vi "BRig_Host_v0,54.vi"() -> ()   [LabVIEW 2014]
uses:
  <vilib>/WebDAVClient/Advanced/SessionHandle.ctl
  BRig_Host__global__stopHost.vi
  <vilib>/Utility/file.llb/Write To Spreadsheet File (DBL).vi
  <vilib>/WebDAVClient/NI_WebDAV.lvlib
panel:
  out "output_dataTS":u16[][](array[numeric])
  out "output_dataPlot":u16[][](array[numeric])
  out "DAB_nTimeout":u16 caption="# Rewards in Current Block"
  out "FreeReward_c_R":u16
  out "FreeReward_c_L":u16
  out "BTPR_avg_R":dbl
  out "T2R_avg_R":dbl
  out "BTPR_avg_L":dbl
  out "T2R_avg_L":dbl
  out "BTPR_cur":u16
  out "T2R_cur":u16
  out "nReward":u16 caption="# Rewards in Current Block"
  out "BUR_target":u16 caption="Target Trials Per Block"
  out "nTrial":u16
  out "nReward_Right":u16 caption="# Rewards Total (Right)"
  out "nReward_Left":u16 caption="# Rewards Total (Left)"
  out "nReward_cur":u16 caption="# Rewards in Current Block"
  out "TpB_target":u16 caption="Target Trials Per Block"
  out "iBlock":u16 caption="Current Block"
  out "iTrial":u16 caption="Current Trial"
  out "DAB_nRewards_ProbLow_percent":u16 caption="# Rewards Total (Right)"
  out "DAB_nRewards_ProbHigh_percent":u16 caption="# Rewards Total (Left)"
  out "DAB_nRewards_ProbLow":u16 caption="# Rewards Total (Right)"
  out "DAB_nRewards_ProbHigh":u16 caption="# Rewards Total (Left)"
  out "DAB_nRewards_total":u16 caption="# Rewards in Current Block"
  out "DAB_nTrial":u16
  out "DAB_nRewards_Right":u16 caption="# Rewards Total (Right)"
  out "DAB_nRewards_Left":u16 caption="# Rewards Total (Left)"
  out "writeError":bool
  out "error IO":errorcluster
  out "error_loopP_loadSettings":errorcluster caption="error out"
  out "testCmdList":u16[][](array[numeric])
  in  "ClosedLoop":bool
  in  "module":string=" module1 "
  in  "input_updateTrial_subsequent":u16
  in  "input_updateTrial_first":u16
  in  "input_forceUpdate":bool
  in  "ClosedLoop":u16[](array[numeric])
  in  "testNewLaserSettings":bool
  in  "LoadSettings":bool
  in  "DisplayNumber":u16
  out "XY Graph":cluster{u16[], u16[]}[](graph)
  in  "threshold_2":u16=600
  in  "threshold_1":u16=300
  in  "Port (F=A/B, T=C)":bool
  out "I_ExpRun":bool
  out "TCP_connection":bool
  in  "stopHost":bool
  # "# Trials Displayed\n( 0 = all )"
  # "Selection\nTime Thresholds"
  # "Dual Armed Bandit"
  # "Standard or 2 Cues"
  # "Total"
  # "# Trials"
  # "# Rewards"
  # "Block Target"
  # "# Blocks"
  # "# Trials"
  # "# Rewards"
  # "Left           Right"
  # "Bad Trials\nPost Reward"
  # "Trials 2 Reward"
  # "# Timeouts"
  # "Block"
  # "# Trials"
  # "# Rewards"
  # "Current\nBlock"
  # "# Selections"
  # "High Prob    Low Prob"
  # "avg L"
  # "Total"
  # "# Rewards"
  # "# Trials"
  # "avg R"
  # "% Selections"
  # "High Prob    Low Prob"
  # "FreeRewards"
  # "Left           Right"
  # "Unknown"
  # "reward1"
  # "reward2"
  # "reward3"
  # "wrong1"
  # "wrong2"
  # "wrong3"
  # "timeout"
  # "trig1"
  # "trig2"
  # "Port Switch\nToggle TRUE if debugging"
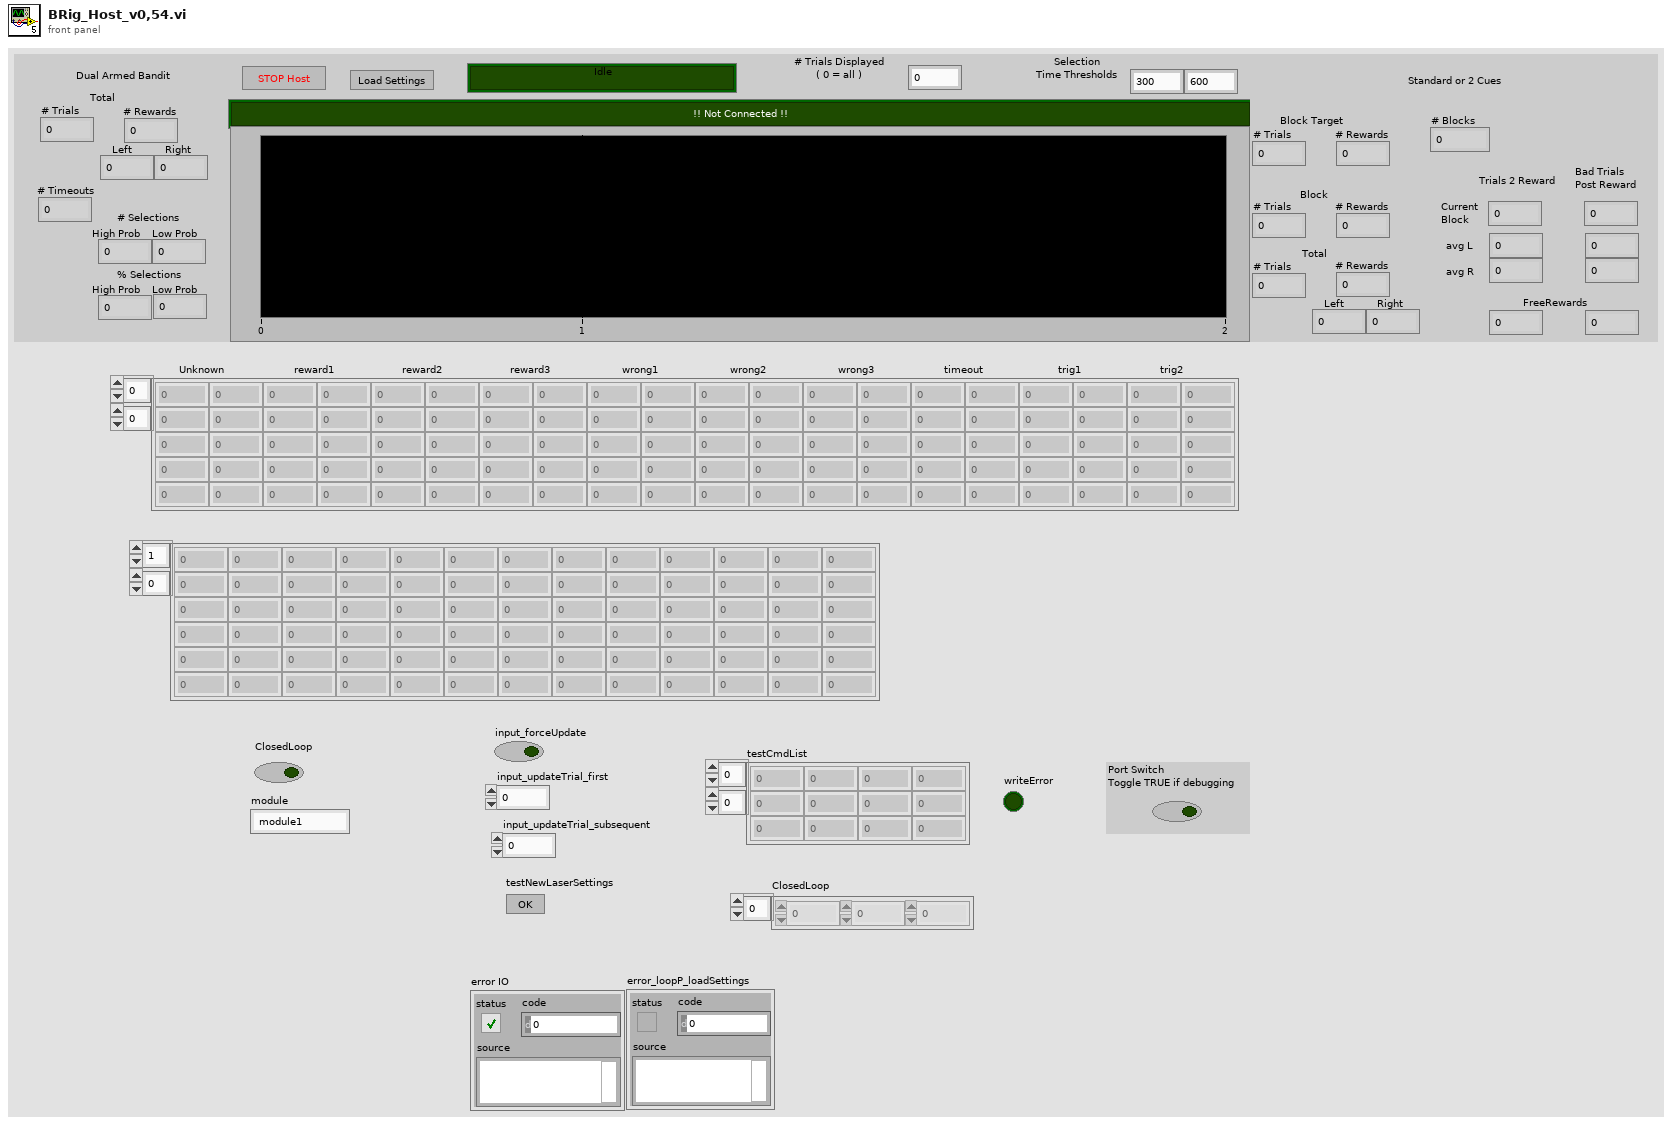
[diagram p1: front panel]
types:
  T1 = typedef "NI_WebDAV.lvlib/SessionHandle.ctl" = refnum<k1>
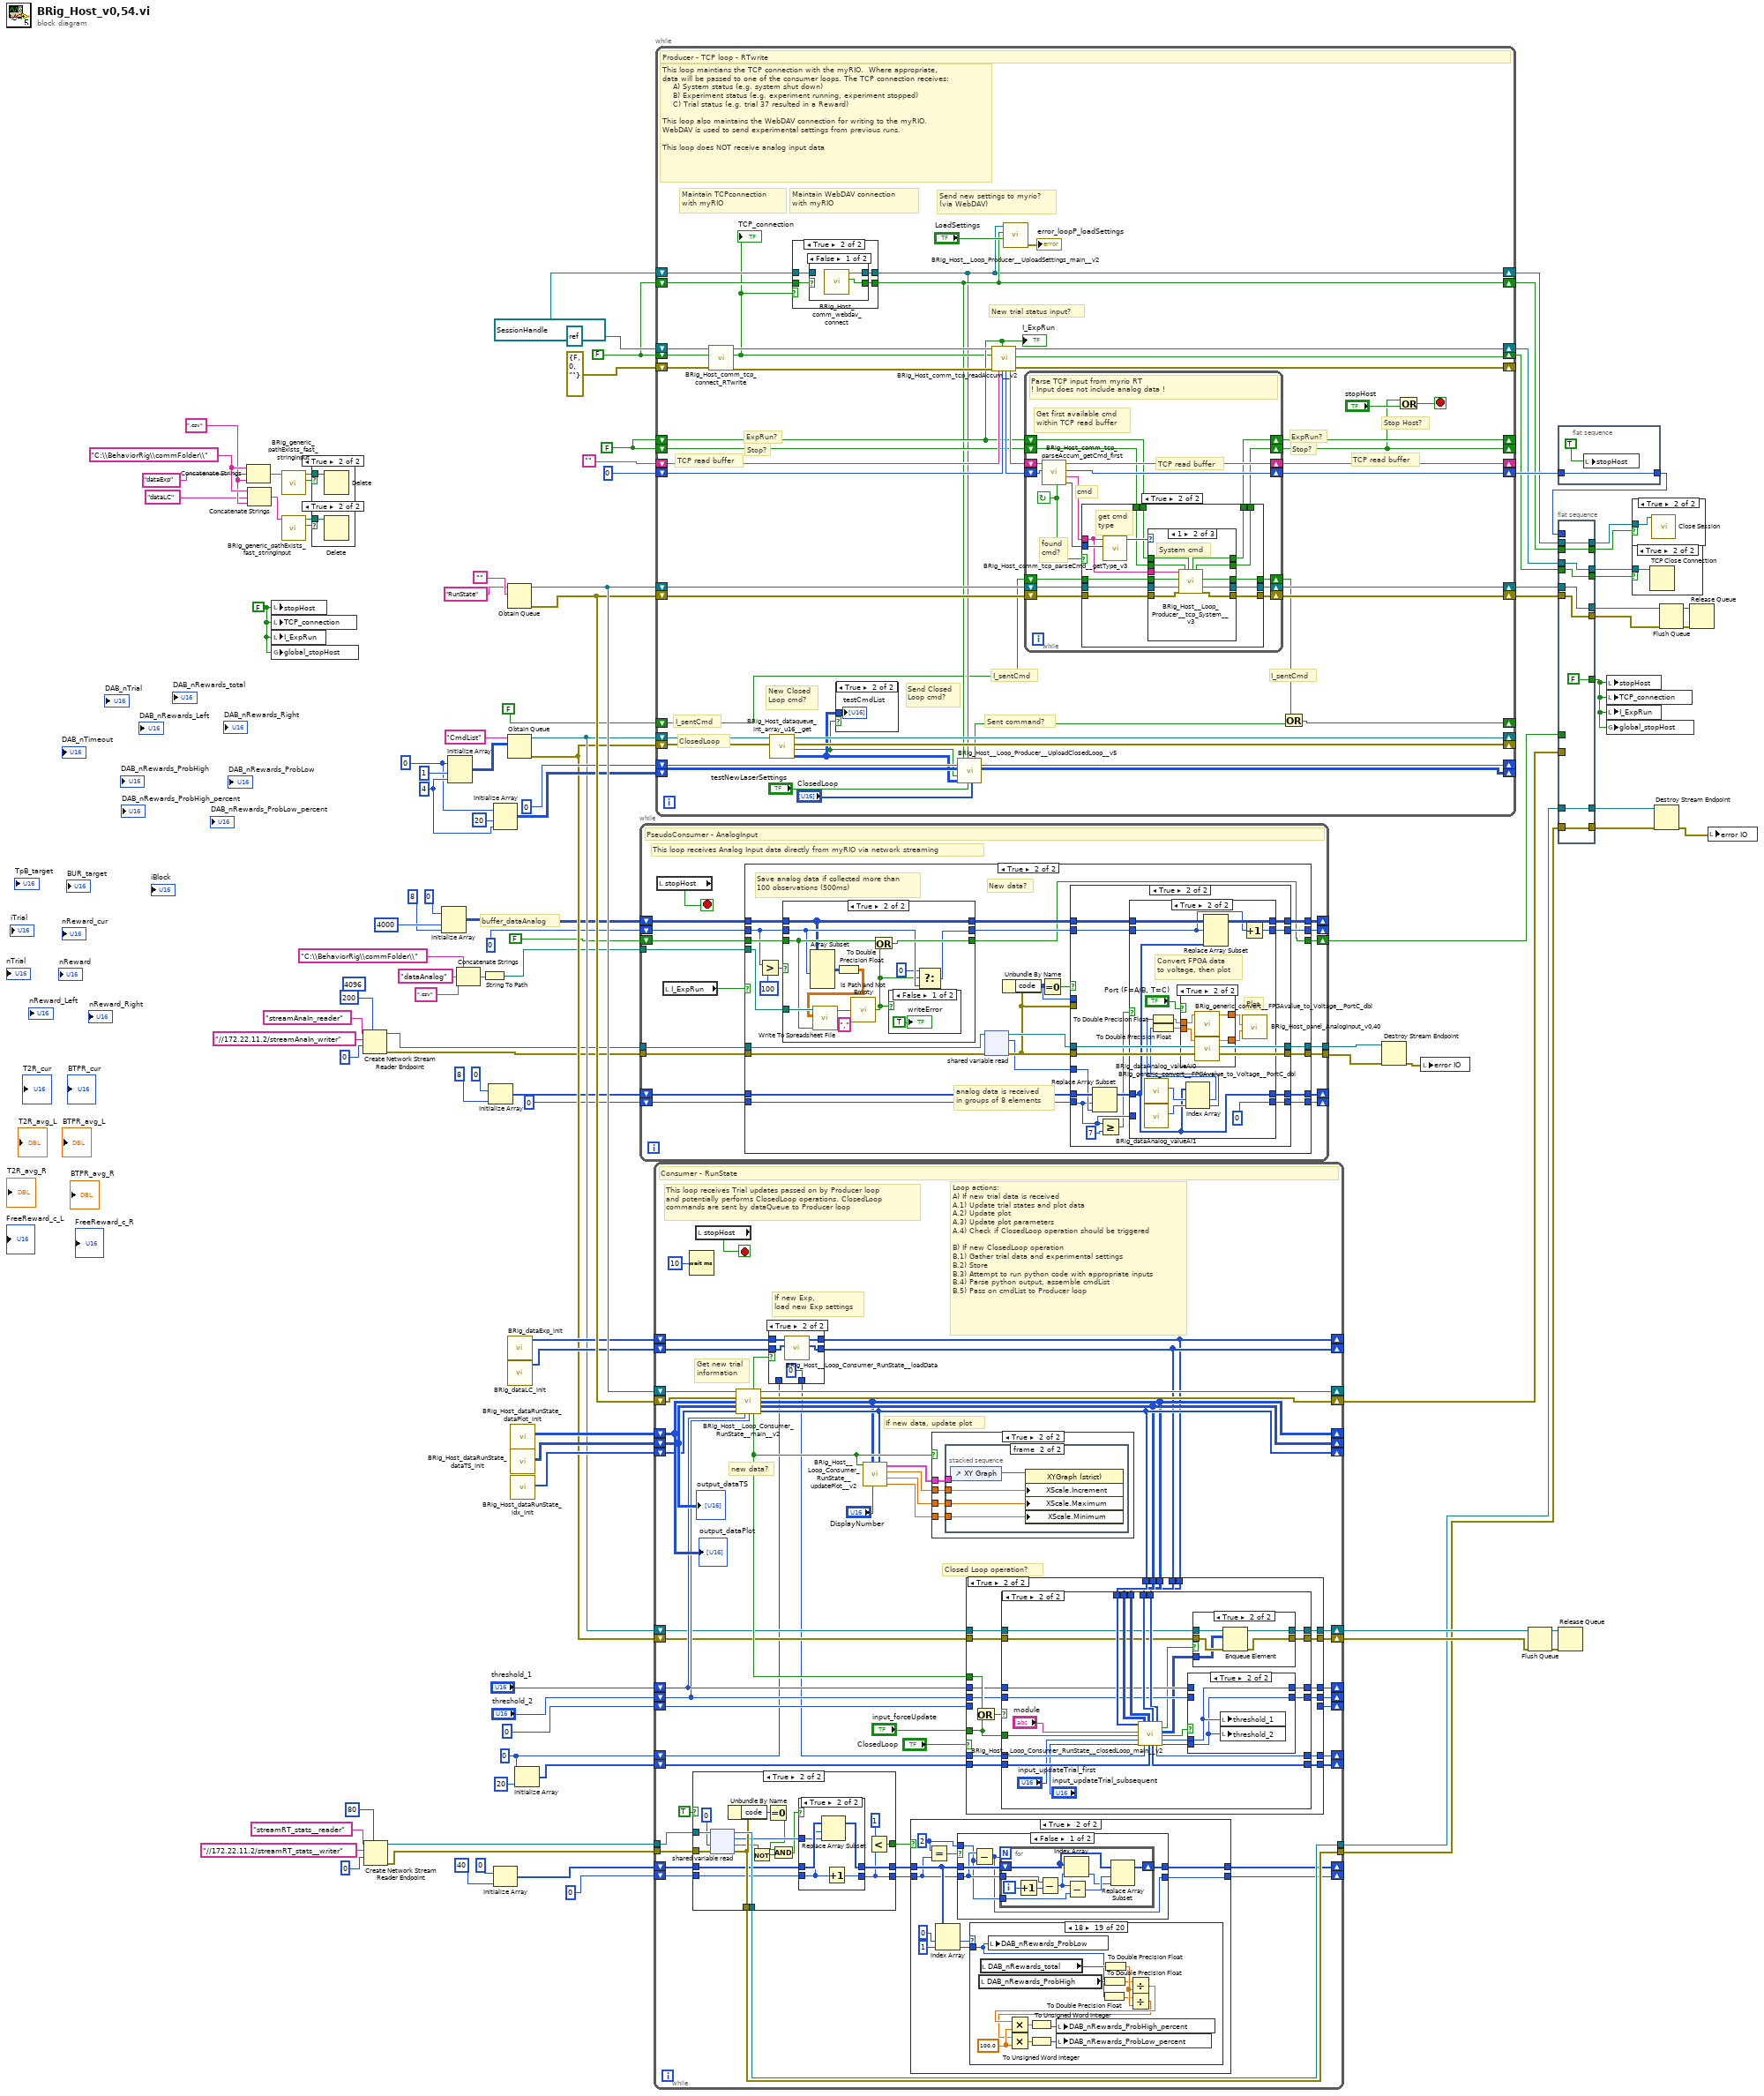
[diagram p0: block diagram]
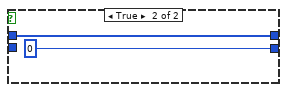
[diagram p9: hidden frame]
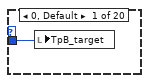
[diagram p10: hidden frame]
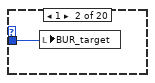
[diagram p11: hidden frame]
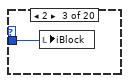
[diagram p12: hidden frame]
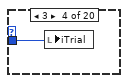
[diagram p13: hidden frame]
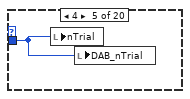
[diagram p14: hidden frame]
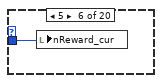
[diagram p15: hidden frame]
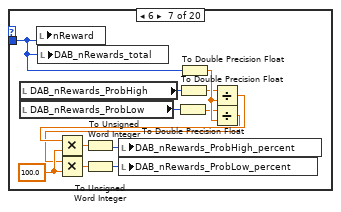
[diagram p16: hidden frame]
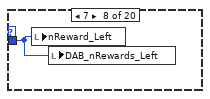
[diagram p17: hidden frame]
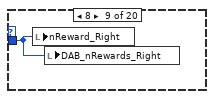
[diagram p18: hidden frame]
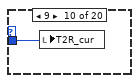
[diagram p19: hidden frame]
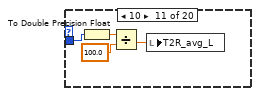
[diagram p20: hidden frame]
diagram:
  (unwired) 4096 ("reader buffer size")
  w41 = u16 0 ("element")
  w42 = 4 ("dimension size")
  w58 = u16 0
  w70 = ".csv" ("string")
  w71 = "C:\\BehaviorRig\\commFolder\\"
  w83 = T1 refnum items=["Session NI_WebDAV"] ("session handle")
  w101 = FALSE ("stopHost")
  w102 = FALSE
  w84 = FALSE
  # "buffer_dataAnalog"
  n1 = Concatenate Strings(w71, "dataExp" ("string"), w70) -> (w65:string)
  n2 = Concatenate Strings(w71, "dataLC" ("string"), w70) -> (w62:string)
  n3 = local write "stopHost"(w101) -> ()
  n4 = local write "TCP_connection"(w101) -> ()
  n5 = local write "I_ExpRun"(w101) -> ()
  n6 = global write "BRig_Host__global__stopHost.vi" "global_stopHost"(w101) -> ()
  n7 = call "BRig_generic_pathExists_fast_stringInput.vi"("input_filePath"=w65) -> ("output_Iexist"=w67:bool, "output_filePath"=w66:path)  [unwired: 8 in, 1 out]
  n8 = call "BRig_generic_pathExists_fast_stringInput.vi"("input_filePath"=w62) -> ("output_Iexist"=w63:bool, "output_filePath"=w64:path)  [unwired: 8 in, 1 out]
  n9 = case shown="True" w67 {
    tunnel: w66 -> [_ w107]
    frame False {
    }
    frame True {
      n10 = Delete(path (use dialog)=w107) -> ()  [unwired: 4 in, 3 out]
    }
  }
  n11 = case shown="True" w63 {
    tunnel: w64 -> [_ w108]
    frame False {
    }
    frame True {
      n12 = Delete(path (use dialog)=w108) -> ()  [unwired: 4 in, 3 out]
    }
  }
  n13 = Create Network Stream Reader Endpoint(7:200 ("reader buffer size"), 9:u16 0 ("element"), 10:"//172.22.11.2/streamAnaIn_writer" ("writer url"), 11:"streamAnaIn_reader" ("reader name")) -> (0:w25:errorcluster, 3:w26:refnum<k21>)  [unwired: 3 in]
  n14 = Create Network Stream Reader Endpoint(7:80 ("reader buffer size"), 9:u16 0 ("element"), 10:"//172.22.11.2/streamRT_stats__writer" ("writer url"), 11:"streamRT_stats__reader" ("reader name")) -> (0:w11:errorcluster, 3:w12:refnum<k21>)  [unwired: 3 in]
  n15 = Initialize Array(u16 0 ("element"), 4000 ("dimension size"), 8 ("dimension size")) -> (w37:u16[][])
  n16 = Initialize Array(w41, 1 ("dimension size"), w42) -> (w53:u16[][])
  n17 = Concatenate Strings("C:\\BehaviorRig\\commFolder\\" ("string"), "dataAnalog" ("input_filename"), ".csv" ("string")) -> (w34:string)
  n18 = String To Path(string=w34) -> (path=w31:path)
  n19 = Initialize Array(u16 0 ("element"), 8 ("dimension size")) -> (w18:u16[])
  n20 = Initialize Array(w41, 20 ("dimension size"), w42) -> (w72:u16[][])
  n21 = Initialize Array(u16 0 ("element"), 40 ("dimension size")) -> (w8:u16[])
  n22 = Obtain Queue(name (unnamed)="RunState", element data type="") -> (queue out=w93:refnum<queue>, error out=w92:errorcluster)  [unwired: 3 in, 1 out]
  n23 = Obtain Queue(name (unnamed)="CmdList", element data type=w53) -> (queue out=w52:refnum<queue>, error out=w51:errorcluster)  [unwired: 3 in, 1 out]
  n24 = call "BRig_dataExp_init.vi"() -> ("output_dataExp"=w61:u16[])  [unwired: 11 in]
  n25 = call "BRig_dataLC_init.vi"() -> ("output_dataLC"=w60:u16[])  [unwired: 11 in]
  n26 = call "BRig_Host_dataRunState_dataPlot_init.vi"() -> ("output_dataPlot"=w89:u16[][])  [unwired: 11 in]
  n27 = call "BRig_Host_dataRunState_dataTS_init.vi"() -> ("output_dataTS"=w88:u16[][])  [unwired: 11 in]
  n28 = call "BRig_Host_dataRunState_idx_init.vi"() -> ("output_idx"=w87:i32[])  [unwired: 11 in]
  n29 = Initialize Array(w58, 20 ("dimension size")) -> (w56:u16[])
  n30 = while {
    shift-right: [w123] -> _
    shift-left: w37 -> [w125]
    shift-right: [w122] -> _
    shift-left: 0 -> [w124]
    tunnel: w31 -> [w121]
    shift-right: [w119] -> w29
    shift-left: FALSE -> [w120]
    tunnel: w26 -> [w117]
    tunnel: w25 -> [w116]
    tunnel: [w115] -> w23
    tunnel: [w114] -> w22
    shift-right: [w111] -> _
    shift-left: w18 -> [w113]
    shift-right: [w110] -> _
    shift-left: 0 ("element") -> [w112]
    stop <- w109 stop-if-true
    # "This loop receives Analog Input data directly from myRIO via network streaming"
    # "PseudoConsumer - AnalogInput"
    n31 = local read "stopHost"() -> (w109:bool)
    n32 = local read "I_ExpRun"() -> (w118:bool)
    n33 = case shown="True" w118 {
      tunnel: w125 -> [w132 w156]
      tunnel: w124 -> [_ w142]
      tunnel: [w132 w151] -> w123
      tunnel: [0 w149] -> w122
      tunnel: w121 -> [_ w154]
      tunnel: w120 -> [_ w155]
      tunnel: [FALSE w139] -> w119
      tunnel: w117 -> [w129 w148]
      tunnel: w116 -> [w128 w147]
      tunnel: [w129 w145] -> w115
      tunnel: [w128 w143] -> w114
      tunnel: w113 -> [w127 w137]
      tunnel: w112 -> [_ w136]
      tunnel: [w127 w135] -> w111
      tunnel: [0 ("element") w134] -> w110
      frame False {
        n34 = Wait (ms)(milliseconds to wait=u32 20) -> ()  [unwired: 1 out]
      }
      frame True {
        # "analog data is received\nin groups of 8 elements"
        # "New data?"
        # "Save analog data if collected more than\n100 observations (500ms)"
        n35 = Greater?(x=w142, y=100) -> (0:w157:bool)
        n36 = case shown="True" w157 {
          tunnel: w156 -> [w216 w219]
          tunnel: [w216 w219] -> w152
          tunnel: w142 -> [w215 w221]
          tunnel: w155 -> [w214 w223]
          tunnel: [w215 w220] -> w150
          tunnel: [w214 w222] -> w139
          tunnel: w154 -> [_ w228]
          frame False {
          }
          frame True {
            n37 = Array Subset(array=w219, length (row)=w221) -> (w227:u16[][])  [unwired: 3 in]
            n38 = To Double Precision Float(number=w227) -> (double precision float=w226:dbl[][])
            n39 = call-poly <vilib>:"Write To Spreadsheet File.vi"("delimiter (\\t)"="," ("delimiter (\\t)"), "append to file? (new file:F)"=w223, "2D data"=w226, "file path (dialog if empty)"=w228) -> ("new file path (Not A Path if cancelled)"=w224:path)  [unwired: 4 in]
            n40 = call <vilib>:"Is Path and Not Empty.vi"("path"=w224) -> ("Is Path and Not Empty?"=w217:bool)  [unwired: 4 in]
            n41 = Or(x=w223, y=w217) -> (x .or. y?=w222:bool)
            n42 = case shown="False" w217 {
              frame False {
                "writeError" <- TRUE ("writeError")
              }
              frame True {
              }
            }
            n43 = Select(t=0, s=w217, f=w221) -> (s? t:f=w220:i32)
          }
        }
        n44 = shared-variable-read(w148, w147) -> (w146:refnum<k21>, w144:errorcluster, w138:u16)  [unwired: 1 in, 1 out]
        n45 = Unbundle By Name(w144) -> ("code"=w140:i32)
        n46 = Equal To 0?(x=w140) -> (x = 0?=w153:bool)
        n47 = case shown="True" w153 {
          tunnel: w152 -> [w170 w185]
          tunnel: [w170 w184] -> w151
          tunnel: w150 -> [w169 w183]
          tunnel: [w169 w182] -> w149
          tunnel: w144 -> [w167 _]
          tunnel: w146 -> [w166 w181]
          tunnel: [w166 w181] -> w145
          tunnel: w144 -> [w165 w180]
          tunnel: [w165 w180] -> w143
          tunnel: w140 -> [w164 _]
          tunnel: w138 -> [_ w178]
          tunnel: w137 -> [w159 w179]
          tunnel: w136 -> [w158 w176]
          tunnel: [w159 w173] -> w135
          tunnel: [w158 w175] -> w134
          frame False {
            n48 = Equal?(x=-314100, y=w164) -> (x = y?=w162:bool)
            n49 = Equal?(x=-314220, y=w164) -> (x = y?=w161:bool)
            n50 = Or(x=w162, y=w161) -> (x .or. y?=w160:bool)
            n51 = case shown="False" w160 {
              tunnel: w167 -> [w171 _]
              frame False {
                "error IO" <- w171
              }
              frame True {
              }
            }
          }
          frame True {
            n52 = Replace Array Subset(array=w179, new element=w178, index=w176) -> (w174:u16[])
            n53 = Greater Or Equal?(x=w176, y=7) -> (x >= y?=w172:bool)
            n54 = case shown="True" w172 {
              tunnel: w185 -> [w190 w205]
              tunnel: [w190 w204] -> w184
              tunnel: w183 -> [w189 w203]
              tunnel: [w189 w202] -> w182
              tunnel: w176 -> [w188 _]
              tunnel: [w187 0 ("y")] -> w175
              tunnel: w174 -> [w186 w193]
              tunnel: [w186 w193] -> w173
              frame False {
                n55 = Increment(x=w188) -> (x+1=w187:i32)
              }
              frame True {
                # "Convert FPGA data\nto voltage, then plot"
                # "Plot"
                n56 = call "BRig_dataAnalog_valueAI0.vi"() -> ("output_valueAI0"=w195:i32)  [unwired: 11 in]
                n57 = call "BRig_dataAnalog_valueAI1.vi"() -> ("output_valueAI1"=w196:i32)  [unwired: 11 in]
                n58 = Index Array(array=w193, index #1=w195, index #2=w196) -> (element #1=w192:u16, element #2=w191:u16)
                n59 = To Double Precision Float(number=w192) -> (double precision float=w197:dbl)
                n60 = To Double Precision Float(number=w191) -> (double precision float=w198:dbl)
                n61 = case shown="True" "Port (F=A/B, T=C)" {
                  tunnel: w197 -> [w207 w213]
                  tunnel: w198 -> [w206 w212]
                  tunnel: [w209 w211] -> w200
                  tunnel: [w208 w210] -> w199
                  frame False {
                    n62 = call "BRig_generic_convert__FPGAvalue_to_Voltage__PortAorB_dbl.vi"("input_FPGAvalue_PortAorB"=w207) -> ("output_voltage"=w209:dbl)  [unwired: 10 in]
                    n63 = call "BRig_generic_convert__FPGAvalue_to_Voltage__PortAorB_dbl.vi"("input_FPGAvalue_PortAorB"=w206) -> ("output_voltage"=w208:dbl)  [unwired: 10 in]
                  }
                  frame True {
                    n64 = call "BRig_generic_convert__FPGAvalue_to_Voltage__PortC_dbl.vi"("input_FPGAvalue_PortC"=w213) -> ("output_voltage"=w211:dbl)  [unwired: 10 in]
                    n65 = call "BRig_generic_convert__FPGAvalue_to_Voltage__PortC_dbl.vi"("input_FPGAvalue_PortC"=w212) -> ("output_voltage"=w210:dbl)  [unwired: 10 in]
                  }
                }
                n66 = Replace Array Subset(array=w205, new element=w193, index (row)=w203) -> (w204:u16[][])  [unwired: 1 in]
                n67 = Increment(x=w203) -> (x+1=w202:i32)
                n68 = call "BRig_Host_panel_AnalogInput_v0,40.vi"("graph_ai1"=w199, "graph_ai0"=w200) -> ()  [unwired: 10 in]
              }
            }
          }
        }
      }
    }
  }
  n69 = while {
    shift-right: [w274] -> _
    shift-left: w93 -> [w275]
    shift-right: [w272] -> w46
    shift-left: w92 -> [w273]
    shift-right: [w255] -> _
    shift-left: w89 -> [w271]
    shift-right: [w256] -> _
    shift-left: w88 -> [w270]
    shift-right: [w257] -> _
    shift-left: w87 -> [w269]
    shift-right: [w265] -> _
    shift-left: "threshold_1" -> [w264]
    shift-right: [w263] -> _
    shift-left: "threshold_2" -> [w262]
    shift-right: [w253] -> _
    shift-left: w61 -> [w267]
    shift-right: [w254] -> _
    shift-left: w60 -> [w266]
    shift-right: [w247] -> _
    shift-left: w58 -> [w245]
    shift-right: [w259] -> _
    shift-left: u8 0 -> [w260]
    shift-right: [w246] -> _
    shift-left: w56 -> [w243]
    shift-right: [w250] -> w48
    shift-left: w52 -> [w252]
    shift-right: [w249] -> w47
    shift-left: w51 -> [w251]
    tunnel: w12 -> [w241]
    tunnel: w11 -> [w240]
    shift-right: [w232] -> _
    shift-left: w8 -> [w237]
    shift-right: [w231] -> _
    shift-left: 0 ("element") -> [w236]
    tunnel: [w239] -> w4
    tunnel: [w238] -> w3
    stop <- w242 stop-if-true
    # "Closed Loop operation?"
    # "Loop actions:\nA) If new trial data is received\nA.1) Update trial states and plot data\nA.2) Update plot\nA.3) Update plot parameters\nA.4) Check if ClosedLoop operation should be triggered\n\nB) If new ClosedLoop operation\nB.1) Gather trial data and experimental settings\nB.2) Store\nB.3) Attempt to run python code with appropriate inputs\nB.4) Parse python output, assemble cmdList\nB.5) Pass on cmdList to Producer loop"
    # "This loop receives Trial updates passed on by Producer loop\nand potentially performs ClosedLoop operations. ClosedLoop\ncommands are sent by dataQueue to Producer loop"
    # "If new data, update plot"
    # "If new Exp,\nload new Exp settings"
    # "new data?"
    # "Get new trial\ninformation"
    # "Consumer - RunState"
    n70 = Wait (ms)(milliseconds to wait=u32 10) -> ()  [unwired: 1 out]
    n71 = case shown="True" TRUE {
      selector: TRUE -> [w282 _]
      tunnel: w241 -> [w286 w302]
      tunnel: w240 -> [w285 w301]
      tunnel: [w286 w300] -> w239
      tunnel: [w285 w299] -> w238
      tunnel: w237 -> [w284 w297]
      tunnel: w236 -> [w283 w296]
      tunnel: [w282 w294] -> w235
      tunnel: [w284 w293] -> w234
      tunnel: [w283 w292] -> w233
      frame False {
      }
      frame True {
        n72 = shared-variable-read(w302, w301, 0 ("timeout ms (-1)")) -> (w300:refnum<k21>, w299:errorcluster, w290:bool, w298:u16)
        n73 = Unbundle By Name(w299) -> ("code"=w303:i32)
        n74 = Not(x=w290) -> (.not. x?=w289:bool)
        n75 = Equal To 0?(x=w303) -> (x = 0?=w288:bool)
        n76 = And(x=w288, y=w289) -> (x .and. y?=w287:bool)
        n77 = case shown="True" w287 {
          tunnel: w298 -> [_ w309]
          tunnel: w297 -> [w305 w310]
          tunnel: w296 -> [w304 w308]
          tunnel: [w305 w306] -> w293
          tunnel: [w304 w307] -> w292
          frame False {
          }
          frame True {
            n78 = Replace Array Subset(array=w310, new element=w309, index=w308) -> (w306:u16[])
            n79 = Increment(x=w308) -> (x+1=w307:i32)
          }
        }
        n80 = Less?(x=1, y=w292) -> (x < y?=w294:bool)
      }
    }
    n81 = local read "stopHost"() -> (w242:bool)
    n82 = call "BRig_Host__Loop_Consumer_RunState__main__v2.vi"("input_hDataQueue"=w275, "input_errorDataQueue"=w273, "input_dataPlot"=w271, "input_dataTS"=w270, "input_idx"=w269, "threshold_1"=w264, "threshold_2"=w262) -> ("output_ExpStart"=w268:bool, "output_hDataQueue"=w274:refnum<queue>, "output_errorDataQueue"=w272:errorcluster, "output_dataPlot"=w255:u16[][], "output_dataTS"=w256:u16[][], "output_updatePlot"=w258:bool, "output_idx"=w257:i32[])  [unwired: 2 in]
    n83 = case shown="True" w268 {
      tunnel: w267 -> [w490 w492]
      tunnel: [w490 w495] -> w253
      tunnel: w266 -> [w489 w493]
      tunnel: [w489 w494] -> w254
      tunnel: w245 -> [w488 _]
      tunnel: [w488 u16 0] -> w244
      frame False {
      }
      frame True {
        n84 = call "BRig_Host__Loop_Consumer_RunState__loadData.vi"("input_dataLC"=w493, "input_dataExp"=w492) -> ("output_dataLC"=w494:u16[], "output_dataExp"=w495:u16[])  [unwired: 8 in]
      }
    }
    n85 = call "BRig_Host__Loop_Consumer_RunState__updatePlot__v2.vi"("input_idx"=w257, "input_DisplayNumber"="DisplayNumber", "input_dataPlot"=w255, "input_updatePlot"=w258) -> ("output_X_min"=w278:dbl, "output_X_max"=w277:dbl, "output_X_inc"=w276:dbl, "XY Graph"=w279:cluster{u16[], u16[]}[])  [unwired: 4 in]
    n86 = case shown="True" w235 {
      tunnel: w234 -> [w312 w317]
      tunnel: w233 -> [w311 w315]
      tunnel: [w312 w316] -> w232
      tunnel: [w311 w314] -> w231
      frame False {
      }
      frame True {
        w313 = 2 ("x")
        n87 = Equal?(x=w313, y=w315) -> (x = y?=w318:bool)
        n88 = Index Array(array=w317, index #1=0 ("index"), index #2=1 ("index")) -> (element #1=w320:u16, element #2=w319:u16)
        n89 = case shown="False" w318 {
          tunnel: w317 -> [w327 w338]
          tunnel: [w323 w338] -> w316
          tunnel: w315 -> [w326 _]
          tunnel: [w324 0 ("index")] -> w314
          tunnel: w313 -> [w325 _]
          frame False {
            n90 = Subtract(x=w326, y=w325) -> (x-y=w324:i32)
            n91 = for {
              N: w324 -> [_]
              shift-right: [w328] -> w323
              shift-left: w327 -> [w331]
              tunnel: w326 -> [w334]
              tunnel: w325 -> [w333]
              i -> [w336]
              n92 = Increment(x=w336) -> (x+1=w335:i32)
              n93 = Subtract(x=w334, y=w335) -> (x-y=w332:i32)
              n94 = Index Array(array=w331, index=w332) -> (element=w329:u16)
              n95 = Subtract(x=w332, y=w333) -> (x-y=w330:i32)
              n96 = Replace Array Subset(array=w331, new element=w329, index=w330) -> (w328:u16[])
            }
          }
          frame True {
          }
        }
        n97 = case shown="18" w320 {
          tunnel: w319 -> [w339 w340 w341 w342 w343 w344 w352 w358 w359 w360 w364 w368 w369 w371 w375 w378 w379 w380 w393 w406]
          frame 0, Default {
            n98 = local write "TpB_target"(w339) -> ()
          }
          frame 1 {
            n99 = local write "BUR_target"(w340) -> ()
          }
          frame 2 {
            n100 = local write "iBlock"(w341) -> ()
          }
          frame 3 {
            n101 = local write "iTrial"(w342) -> ()
          }
          frame 4 {
            n102 = local write "nTrial"(w343) -> ()
            n103 = local write "DAB_nTrial"(w343) -> ()
          }
          frame 5 {
            n104 = local write "nReward_cur"(w344) -> ()
          }
          frame 6 {
            w351 = 100.0 ("y")
            n105 = local read "DAB_nRewards_ProbHigh"() -> (w353:u16)
            n106 = local read "DAB_nRewards_ProbLow"() -> (w354:u16)
            n107 = local write "nReward"(w352) -> ()
            n108 = local write "DAB_nRewards_total"(w352) -> ()
            n109 = To Double Precision Float(number=w354) -> (double precision float=w356:dbl)
            n110 = To Double Precision Float(number=w353) -> (double precision float=w355:dbl)
            n111 = To Double Precision Float(number=w352) -> (double precision float=w357:dbl)
            n112 = Divide(x=w355, y=w357) -> (x/y=w350:dbl)
            n113 = Multiply(x=w350, y=w351) -> (x*y=w348:dbl)
            n114 = To Unsigned Word Integer(number=w348) -> (unsigned 16bit integer=w346:u16)
            n115 = local write "DAB_nRewards_ProbHigh_percent"(w346) -> ()
            n116 = Divide(x=w356, y=w357) -> (x/y=w349:dbl)
            n117 = Multiply(x=w349, y=w351) -> (x*y=w347:dbl)
            n118 = To Unsigned Word Integer(number=w347) -> (unsigned 16bit integer=w345:u16)
            n119 = local write "DAB_nRewards_ProbLow_percent"(w345) -> ()
          }
          frame 7 {
            n120 = local write "nReward_Left"(w358) -> ()
            n121 = local write "DAB_nRewards_Left"(w358) -> ()
          }
          frame 8 {
            n122 = local write "nReward_Right"(w359) -> ()
            n123 = local write "DAB_nRewards_Right"(w359) -> ()
          }
          frame 9 {
            n124 = local write "T2R_cur"(w360) -> ()
          }
          frame 10 {
            n125 = To Double Precision Float(number=w364) -> (double precision float=w363:dbl)
            n126 = Divide(x=w363, y=100.0) -> (x/y=w361:dbl)
            n127 = local write "T2R_avg_L"(w361) -> ()
          }
          frame 11 {
            n128 = To Double Precision Float(number=w368) -> (double precision float=w367:dbl)
            n129 = Divide(x=w367, y=100.0) -> (x/y=w365:dbl)
            n130 = local write "T2R_avg_R"(w365) -> ()
          }
          frame 12 {
            n131 = local write "BTPR_cur"(w369) -> ()
          }
          frame 13 {
            n132 = To Double Precision Float(number=w371) -> (double precision float=w373:dbl)
            n133 = Divide(x=w373, y=100.0) -> (x/y=w370:dbl)
            n134 = local write "BTPR_avg_L"(w370) -> ()
          }
          frame 14 {
            n135 = To Double Precision Float(number=w375) -> (double precision float=w376:dbl)
            n136 = Divide(x=w376, y=100.0) -> (x/y=w374:dbl)
            n137 = local write "BTPR_avg_R"(w374) -> ()
          }
          frame 15 {
            n138 = local write "FreeReward_c_L"(w378) -> ()
          }
          frame 16 {
            n139 = local write "FreeReward_c_R"(w379) -> ()
          }
          frame 17 {
            w388 = 100.0 ("y")
            n140 = local read "DAB_nRewards_ProbLow"() -> (w389:u16)
            n141 = local read "DAB_nRewards_total"() -> (w381:u16)
            n142 = local write "DAB_nRewards_ProbHigh"(w380) -> ()
            n143 = To Double Precision Float(number=w389) -> (double precision float=w391:dbl)
            n144 = To Double Precision Float(number=w380) -> (double precision float=w390:dbl)
            n145 = To Double Precision Float(number=w381) -> (double precision float=w392:dbl)
            n146 = Divide(x=w390, y=w392) -> (x/y=w387:dbl)
            n147 = Multiply(x=w387, y=w388) -> (x*y=w385:dbl)
            n148 = To Unsigned Word Integer(number=w385) -> (unsigned 16bit integer=w383:u16)
            n149 = local write "DAB_nRewards_ProbHigh_percent"(w383) -> ()
            n150 = Divide(x=w391, y=w392) -> (x/y=w386:dbl)
            n151 = Multiply(x=w386, y=w388) -> (x*y=w384:dbl)
            n152 = To Unsigned Word Integer(number=w384) -> (unsigned 16bit integer=w382:u16)
            n153 = local write "DAB_nRewards_ProbLow_percent"(w382) -> ()
          }
          frame 18 {
            w401 = 100.0 ("y")
            n154 = local read "DAB_nRewards_ProbHigh"() -> (w402:u16)
            n155 = local read "DAB_nRewards_total"() -> (w394:u16)
            n156 = local write "DAB_nRewards_ProbLow"(w393) -> ()
            n157 = To Double Precision Float(number=w393) -> (double precision float=w404:dbl)
            n158 = To Double Precision Float(number=w402) -> (double precision float=w403:dbl)
            n159 = To Double Precision Float(number=w394) -> (double precision float=w405:dbl)
            n160 = Divide(x=w403, y=w405) -> (x/y=w400:dbl)
            n161 = Multiply(x=w400, y=w401) -> (x*y=w398:dbl)
            n162 = To Unsigned Word Integer(number=w398) -> (unsigned 16bit integer=w396:u16)
            n163 = local write "DAB_nRewards_ProbHigh_percent"(w396) -> ()
            n164 = Divide(x=w404, y=w405) -> (x/y=w399:dbl)
            n165 = Multiply(x=w399, y=w401) -> (x*y=w397:dbl)
            n166 = To Unsigned Word Integer(number=w397) -> (unsigned 16bit integer=w395:u16)
            n167 = local write "DAB_nRewards_ProbLow_percent"(w395) -> ()
          }
          frame 19 {
            n168 = local write "DAB_nTimeout"(w406) -> ()
          }
        }
      }
    }
    n169 = case shown="True" w258 {
      tunnel: w279 -> [_ w499]
      tunnel: w278 -> [_ w498]
      tunnel: w277 -> [_ w497]
      tunnel: w276 -> [_ w496]
      frame False {
      }
      frame True {
        n170 = stacked-sequence {
          tunnel: w499 -> [w500 _]
          tunnel: w498 -> [_ w503]
          tunnel: w497 -> [_ w502]
          tunnel: w496 -> [_ w501]
          frame #0 {
            "XY Graph" <- w500
          }
          frame #1 {
            n171 = control-ref of="XY Graph"() -> (w504:refnum<vi>)
            n172 = property class="XYGraph (strict)"(reference=w504, "XScale.Increment"=w501, "XScale.Maximum"=w502, "XScale.Minimum"=w503) -> ()  [unwired: 1 in, 2 out]
          }
        }
      }
    }
    n173 = case shown="True" "ClosedLoop" {
      tunnel: [w414 w437] -> w265
      tunnel: w264 -> [w415 w438]
      tunnel: [w413 w435] -> w263
      tunnel: w262 -> [w416 w436]
      tunnel: w260 -> [w419 _]
      tunnel: [w412 _] -> w259
      tunnel: w244 -> [w410 w442]
      tunnel: [w410 w440] -> w247
      tunnel: w243 -> [w409 w441]
      tunnel: [w409 w439] -> w246
      tunnel: w258 -> [_ w444]
      tunnel: w257 -> [_ w434]
      tunnel: w256 -> [_ w433]
      tunnel: w255 -> [_ w432]
      tunnel: w254 -> [_ w431]
      tunnel: w253 -> [_ w430]
      tunnel: w252 -> [w408 w429]
      tunnel: w251 -> [w407 w428]
      tunnel: [w408 w427] -> w250
      tunnel: [w407 w426] -> w249
      tunnel: "input_forceUpdate" -> [_ w425]
      frame False {
        n174 = Increment(x=w419) -> (x+1=w411:u8)
        n175 = Less?(x=w411, y=u8 10) -> (x < y?=w417:bool)
        n176 = case shown="False" w417 {
          tunnel: w416 -> [_ w423]
          tunnel: w415 -> [_ w424]
          tunnel: [w421 w424] -> w414
          tunnel: [w420 w423] -> w413
          tunnel: [_ w422] -> w412
          tunnel: w411 -> [_ w422]
          frame False {
            n177 = local read "threshold_1"() -> (w421:u16)
            n178 = local read "threshold_2"() -> (w420:u16)
          }
          frame True {
          }
        }
      }
      frame True {
        n179 = Or(x=w444, y=w425) -> (x .or. y?=w443:bool)
        n180 = case shown="True" w443 {
          tunnel: w425 -> [_ w473]
          tunnel: w442 -> [w450 w476]
          tunnel: w441 -> [w449 w475]
          tunnel: [w450 w469] -> w440
          tunnel: [w449 w470] -> w439
          tunnel: w438 -> [w448 w463]
          tunnel: [w448 w459] -> w437
          tunnel: w436 -> [w447 w462]
          tunnel: [w447 w458] -> w435
          tunnel: w434 -> [_ w468]
          tunnel: w433 -> [_ w467]
          tunnel: w432 -> [_ w466]
          tunnel: w431 -> [_ w465]
          tunnel: w430 -> [_ w464]
          tunnel: w429 -> [w446 w456]
          tunnel: w428 -> [w445 w454]
          tunnel: [w446 w455] -> w427
          tunnel: [w445 w453] -> w426
          frame False {
          }
          frame True {
            n181 = call "BRig_Host__Loop_Consumer_RunState__closedLoop_main__v2.vi"("input_idx"=w468, "input_module"="module", "input_forceUpdate"=w473, "input_updateTrial_first"="input_updateTrial_first", "input_updateTrial_subsequent"="input_updateTrial_subsequent", "input_dataTS"=w467, "input_updateID"=w476, "input_dataPlot"=w466, "input_trialList"=w475, "input_dataLC"=w465, "input_dataExp"=w464) -> ("output_trialList"=w470:u16[], "output_updateID"=w469:u16, 15:"output_cmdList"=w451:bool, 16:"output_cmdList"=w452:u16[][], "output_thres"=w457:bool, "output_thres1"=w461:u16, "output_thres2"=w460:u16)  [unwired: 2 in]
            n182 = case shown="True" w457 {
              tunnel: w463 -> [w485 _]
              tunnel: w462 -> [w484 _]
              tunnel: w461 -> [_ w487]
              tunnel: w460 -> [_ w486]
              tunnel: [w485 w487] -> w459
              tunnel: [w484 w486] -> w458
              frame False {
              }
              frame True {
                n183 = local write "threshold_1"(w487) -> ()
                n184 = local write "threshold_2"(w486) -> ()
              }
            }
            n185 = case shown="True" w451 {
              tunnel: w456 -> [w478 w483]
              tunnel: [w478 w480] -> w455
              tunnel: w454 -> [w477 w482]
              tunnel: [w477 w479] -> w453
              tunnel: w452 -> [_ w481]
              frame False {
              }
              frame True {
                n186 = Enqueue Element(queue=w483, element=w481, error in (no error)=w482) -> (queue out=w480:refnum<queue>, error out=w479:errorcluster)  [unwired: 1 in, 1 out]
              }
            }
          }
        }
      }
    }
    "output_dataPlot" <- w271
    "output_dataTS" <- w270
  }
  n187 = while {
    shift-right: [w531] -> w77
    shift-left: w84 -> [w551]
    shift-right: [w546] -> w78
    shift-left: refnum<k5> refnum ("output_hTCP") -> [w550]
    shift-right: [w545] -> _
    shift-left: errorcluster {"status"=FALSE, "code"=0, "source"=""} ("output_error") -> [w549]
    shift-right: [w540] -> _
    shift-left: "" ("input_strAccum") -> [w544]
    shift-right: [w539] -> w91
    shift-left: 0 ("input_count") -> [w543]
    shift-right: [w538] -> _
    shift-left: w102 -> [w516]
    shift-right: [w514] -> _
    shift-left: w102 -> [w536]
    shift-right: [w533] -> w97
    shift-left: w93 -> [w535]
    shift-right: [w532] -> w96
    shift-left: w92 -> [w534]
    shift-right: [w511] -> w82
    shift-left: w84 -> [w530]
    shift-right: [w510] -> w81
    shift-left: w83 -> [w529]
    shift-right: [w521] -> _
    shift-left: w72 -> [w522]
    shift-right: [w505] -> _
    shift-left: 0 -> [w523]
    shift-right: [w525] -> _
    shift-left: w52 -> [w527]
    shift-right: [w524] -> _
    shift-left: w51 -> [w526]
    shift-right: [w506] -> _
    shift-left: FALSE -> [w509]
    stop <- w513 stop-if-true
    # "ClosedLoop"
    # "TCP read buffer"
    # "TCP read buffer"
    # "I_sentCmd"
    # "Sent command?"
    # "I_sentCmd"
    # "I_sentCmd"
    # "Stop Host?"
    # "Send Closed\nLoop cmd?"
    # "New Closed\nLoop cmd?"
    # "New trial status input?"
    # "ExpRun?"
    # "Stop?"
    # "This loop maintians the TCP connection with the myRIO.  Where appropriate,\ndata will be passed to one of the consumer loops. The TCP connection receives:\n    A) System status (e.g. system shut down)\n    B) Experiment status (e.g. experiment running, experiment stopped)\n    C) Trial status (e.g. trial 37 resulted in a Reward)\n\nThis loop also maintains the WebDAV connection for writing to the myRIO.\nWebDAV is used to send experimental settings from previous runs.\n\nThis loop does NOT receive analog input data"
    # "Send new settings to myrio?\n(via WebDAV)"
    # "ExpRun?"
    # "Stop?"
    # "Maintain TCPconnection\nwith myRIO"
    # "Maintain WebDAV connection\nwith myRIO"
    # "Producer - TCP loop - RTwrite"
    n188 = call "BRig_Host_comm_tcp_connect_RTwrite.vi"("input_error"=w549, "input_connected"=w551, "input_hTCP"=w550) -> ("output_error"=w547:errorcluster, "output_connected"=w515:bool, "output_hTCP"=w548:refnum<k5>)  [unwired: 5 in, 1 out]
    "TCP_connection" <- w515
    n189 = call "BRig_Host_dataqueue_int_array_u16__get.vi"("input_erroDataQueue"=w526, "input_hDataQueue"=w527) -> (0:"output_data"=w518:u16[][], 1:"output_data"=w517:bool, "output_errorDataQueue"=w524:errorcluster, "output_hDataQueue"=w525:refnum<queue>)  [unwired: 6 in]
    n190 = case shown="True" w515 {
      tunnel: w530 -> [w556 w564]
      tunnel: [w555 w563] -> w511
      tunnel: w529 -> [w554 w562]
      tunnel: [w553 w561] -> w510
      frame False {
        n191 = case shown="True" w556 {
          selector: w556 -> [w558 _]
          tunnel: [w558 FALSE] -> w555
          tunnel: w554 -> [w557 w559]
          tunnel: [w557 _] -> w553
          frame False {
          }
          frame True {
            n192 = call <vilib>:"Close Session.vi"("session handle"=w559) -> ()  [unwired: 14 in, 1 out]
          }
        }
      }
      frame True {
        n193 = case shown="False" w564 {
          selector: w564 -> [_ w568]
          tunnel: [w565 w568] -> w563
          tunnel: w562 -> [_ w567]
          tunnel: [w566 w567] -> w561
          frame False {
            n194 = call "BRig_Host_comm_webdav_connect.vi"() -> ("output_Iconnected"=w565:bool, "output_hSession"=w566:T1)  [unwired: 9 in, 1 out]
          }
          frame True {
          }
        }
      }
    }
    n195 = case shown="True" w517 {
      tunnel: w518 -> [_ w552]
      frame False {
      }
      frame True {
        "testCmdList" <- w552
      }
    }
    n196 = call "BRig_Host__Loop_Producer__UploadClosedLoop__v5.vi"("input_arrayBuffer_length"=w523, "input_arrayBuffer"=w522, 4:"input_cmdList"=w517, 5:"input_cmdList"=w518, "input_webdav_status"=w511, "session handle"=w510, "testNewLaserSettings"="testNewLaserSettings", "input_array_LaserSettings"="ClosedLoop") -> ("Sent"=w507:bool, "output_arrayBuffer_length"=w505:i32, "output_arrayBuffer"=w521:u16[][])  [unwired: 9 in]
    n197 = call "BRig_Host_comm_tcp_readAccum__v2.vi"("input_handle_TCP"=w548, "input_connected"=w515, "input_error"=w547, "input_strAccum"=w544, "input_I_ExpRun"=w516, "input_count"=w543) -> ("output_count"=w541:i32, "output_strAccum"=w542:string, "output_handle_TCP"=w546:refnum<k5>, "output_connected"=w531:bool, "output_error"=w545:errorcluster)  [unwired: 9 in]
    n198 = call "BRig_Host__Loop_Producer__UploadSettings_main__v2.vi"("input_LoadSettings"="LoadSettings", "input_webdav_status"=w511, "session handle"=w510) -> ("error out"=→"error_loopP_loadSettings":errorcluster)  [unwired: 8 in]
    n199 = while {
      shift-right: [w582] -> w540
      shift-left: w542 -> [w585]
      shift-right: [w581] -> w539
      shift-left: w541 -> [w584]
      shift-right: [w577] -> w538
      shift-left: w516 -> [w578]
      shift-right: [w575] -> w514
      shift-left: w536 -> [w576]
      shift-right: [w571] -> w533
      shift-left: w535 -> [w574]
      shift-right: [w572] -> w532
      shift-left: w534 -> [w573]
      shift-right: [w569] -> w508
      shift-left: w509 -> [w570]
      stop <- w583 continue-if-true
      # "found\ncmd?"
      # "TCP read buffer"
      # "cmd"
      # "Get first available cmd\nwithin TCP read buffer"
      # "Parse TCP input from myrio RT\n! Input does not include analog data !"
      n200 = call "BRig_Host_comm_tcp_parseAccum_getCmd_first.vi"("input_count"=w584, "input_strAccum"=w585) -> ("output_countCmd"=w579:i32, "output_strCmd"=w580:string, "output_count"=w581:i32, "output_strAccum"=w582:string, "output_I_cmd"=w583:bool)  [unwired: 5 in]
      n201 = case shown="True" w583 {
        tunnel: w580 -> [_ w601]
        tunnel: w579 -> [_ w603]
        tunnel: w578 -> [w590 w596]
        tunnel: [w590 w594] -> w577
        tunnel: w576 -> [w589 w595]
        tunnel: [w589 w593] -> w575
        tunnel: w574 -> [w588 w600]
        tunnel: w573 -> [w587 w599]
        tunnel: [w587 w598] -> w572
        tunnel: [w588 w597] -> w571
        tunnel: w570 -> [w586 w592]
        tunnel: [w586 w591] -> w569
        frame False {
        }
        frame True {
          # "get cmd\ntype"
          n202 = call "BRig_Host_comm_tcp_parseCmd__getType_v3.vi"("input_strCmd"=w601, "input_countCmd"=w603) -> ("output_strType"=w602:u8)  [unwired: 17 in]
          n203 = case shown="1" w602 {
            tunnel: w601 -> [_ w615 w627]
            tunnel: w600 -> [w608 w618 w626]
            tunnel: w599 -> [w607 w619 w625]
            tunnel: [w607 w617 w624] -> w598
            tunnel: [w608 w616 w623] -> w597
            tunnel: w596 -> [w606 w614 w622]
            tunnel: w595 -> [w605 w613 w621]
            tunnel: [w606 w612 w622] -> w594
            tunnel: [w605 w611 w621] -> w593
            tunnel: w592 -> [w604 w610 w620]
            tunnel: [w604 w609 w620] -> w591
            frame 0, Default {
              # "unknown cmd"
            }
            frame 1 {
              # "System cmd"
              n204 = call "BRig_Host__Loop_Producer__tcp_System__v3.vi"("input_strCmd"=w615, "input_I_SentCmd"=w610, "input_hDataQueue"=w618, "input_error_dataqueue"=w619, "input_I_Stop"=w613, "input_I_ExpRun"=w614) -> ("output_I_ExpRun"=w612:bool, "output_I_Stop"=w611:bool, "output_I_sentCmd"=w609:bool, "output_hDataQueue"=w616:refnum<queue>, "output_error"=w617:errorcluster)  [unwired: 9 in]
            }
            frame 2 {
              # "Send to\nconsumer loop"
              # "Trial state cmd"
              n205 = Enqueue Element(queue=w626, element=w627, error in (no error)=w625) -> (queue out=w623:refnum<queue>, error out=w624:errorcluster)  [unwired: 1 in, 1 out]
            }
          }
        }
      }
    }
    n206 = Or(x=w508, y=w507) -> (x .or. y?=w506:bool)
    n207 = Or(x=w514, y="stopHost") -> (x .or. y?=w513:bool)
    "I_ExpRun" <- w516
  }
  n208 = Destroy Stream Endpoint(8:w22, 11:w23) -> (0:w1:errorcluster)
  n209 = local write "error IO"(w1) -> ()
  n210 = Flush Queue(queue=w48, error in (no error)=w47) -> (queue out=w50:refnum<queue>, error out=w49:errorcluster)  [unwired: 1 out]
  n211 = flat-sequence {
    tunnel: w91 -> [w629]
    tunnel: [w629] -> w90
    frame #0 {
      n212 = local write "stopHost"(TRUE ("global_stopHost")) -> ()
    }
  }
  n213 = flat-sequence {
    tunnel: [FALSE] -> w100
    tunnel: w97 -> [w637]
    tunnel: w96 -> [w636]
    tunnel: [w637] -> w95
    tunnel: [w636] -> w94
    tunnel: w90 -> [_]
    tunnel: w82 -> [w634]
    tunnel: w81 -> [w635]
    tunnel: [w635] -> w79
    tunnel: [w634] -> w80
    tunnel: w78 -> [w632]
    tunnel: w77 -> [w633]
    tunnel: [w633] -> w76
    tunnel: [w632] -> w75
    tunnel: w46 -> [_]
    tunnel: w29 -> [_]
    tunnel: [w630] -> w6
    tunnel: [w631] -> w5
    tunnel: w4 -> [w631]
    tunnel: w3 -> [w630]
    frame #0 {
    }
  }
  n214 = Release Queue(queue=w50, error in (no error)=w49) -> ()  [unwired: 1 in, 3 out]
  n215 = local write "stopHost"(w100) -> ()
  n216 = local write "TCP_connection"(w100) -> ()
  n217 = local write "I_ExpRun"(w100) -> ()
  n218 = global write "BRig_Host__global__stopHost.vi" "global_stopHost"(w100) -> ()
  n219 = case shown="True" w80 {
    tunnel: w79 -> [_ w639]
    frame False {
    }
    frame True {
      n220 = call <vilib>:"Close Session.vi"("session handle"=w639) -> ()  [unwired: 14 in, 1 out]
    }
  }
  n221 = case shown="True" w76 {
    tunnel: w75 -> [_ w640]
    frame False {
    }
    frame True {
      n222 = TCP Close Connection(connection ID=w640) -> ()  [unwired: 2 in, 2 out]
    }
  }
  n223 = Destroy Stream Endpoint(8:w6, 11:w5) -> (0:w2:errorcluster)
  n224 = Flush Queue(queue=w95, error in (no error)=w94) -> (queue out=w45:refnum<queue>, error out=w44:errorcluster)  [unwired: 1 out]
  n225 = Release Queue(queue=w45, error in (no error)=w44) -> ()  [unwired: 1 in, 3 out]
  n226 = local write "error IO"(w2) -> ()
